vi "LM_I_27_07_16.vi"   [LabVIEW 2015]
uses:
  <vilib>/NXT/Block Support/NXT_MessageMailbox.ctl
  <vilib>/NXT/Block Support/NXT_OutputPort.ctl
  <vilib>/NXT/Subs/MotorOutput.ctl
  <vilib>/NXT/Block Support/NXT_InputPort.ctl
  <vilib>/NXT/Block Support/NXT_TimerIndex.ctl
  <vilib>/NXT/Dual Mode Library/Advanced/NXTFlag_Assign.vi
  <vilib>/NXT/NXTIO Xnodes/NXTIONodeSubVIs/NXTMoveMotors.vi
  <vilib>/NXT/NXTIO Xnodes/NXTIONodeSubVIs/NXTStopMotors.vi
  <vilib>/NXT/Dual Mode Library/BT/BlueTooth_Write_String.vi
  <vilib>/NXT/Subs/LVHSConnector.ctl
  <vilib>/NXT/NXTIO Xnodes/AddressXNode/NXTIOAddress.xnode
  <vilib>/NXT/NXTIO Xnodes/NXTIOXNode/NXTIO.xnode
  <vilib>/NXT/LegoClasses/BrickReference/BrickReference.lvclass
types:
  T1 = typedef "NXT_MessageMailbox.ctl" = u8
  T2 = typedef "LVHSConnector.ctl" = refnum<class "BrickReference.lvclass">
  T3 = typedef "NXT_InputPort.ctl" = u32
  T4 = typedef "NXT_OutputPort.ctl" = u8
  T5 = typedef "NXT_TimerIndex.ctl" = u8
  T6 = typedef "MotorOutput.ctl" = u8
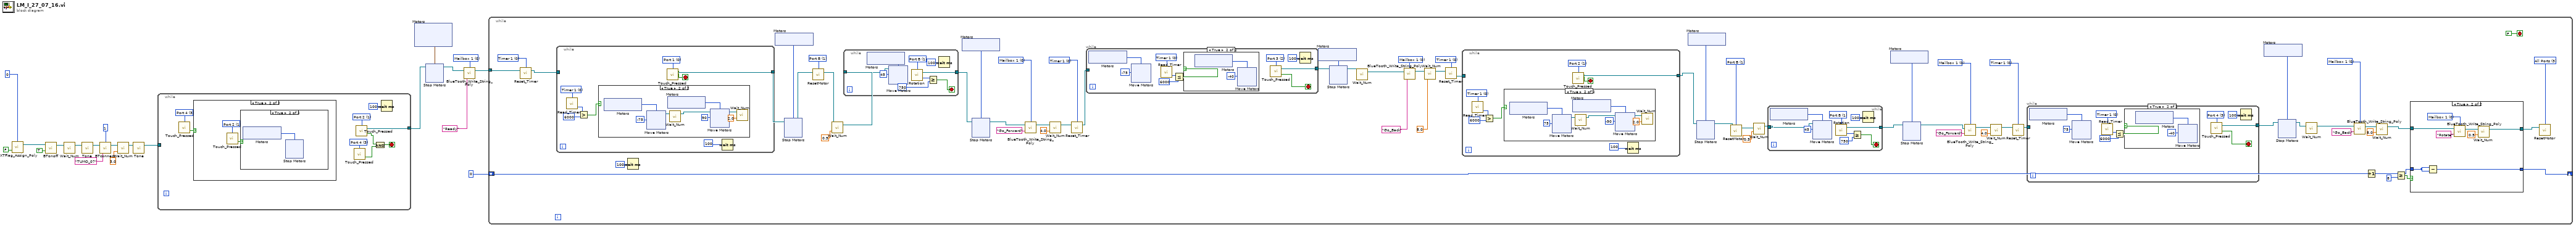
[diagram p0: block diagram]
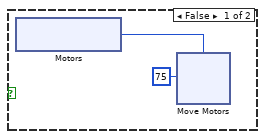
[diagram p2: hidden frame]
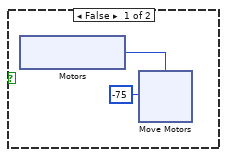
[diagram p3: hidden frame]
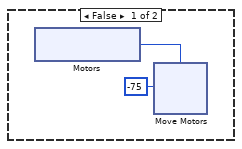
[diagram p4: hidden frame]
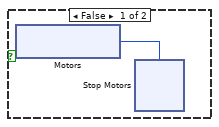
[diagram p5: hidden frame]
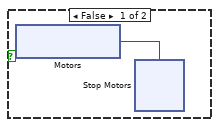
[diagram p7: hidden frame]
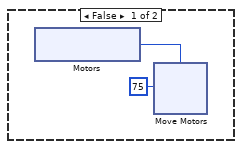
[diagram p8: hidden frame]
diagram:
  w8 = T1 0 items=["Mailbox 1", "Mailbox 2", "Mailbox 3", "Mailbox 4", "Mailbox 5", "Mailbox 6", "Mailbox 7", "Mailbox 8", "Mailbox 9", "Mailbox 10"] ("Mailbox")
  n1 = call-poly <vilib>:"NXTFlag_Assign_Poly.vi"("Flag State"=FALSE, "NXT/EV3 Flag Number"=i8 0) -> ("NXT/EV3"=w4:T2)  [unwired: 2 in]
  n2 = call <vilib>:"BTonoff.vi"("On/Off"=TRUE, "NXT/EV3"=w4) -> ("NXT/EV3"=w13:T2)  [unwired: 1 in, 1 out]
  n3 = call <vilib>:"Wait_Num.vi"("NXT/EV3"=w13) -> ("NXT/EV3"=w12:T2)  [unwired: 3 in]
  n4 = call <vilib>:"Tone.vi"("NXT/EV3"=w12) -> ("NXT/EV3"=w11:T2)  [unwired: 3 in]
  n5 = call <vilib>:"BTconnect.vi"("Partner Name"="TUMO_07", "NXT/EV3"=w11, "Connection"=u8 1) -> ("NXT/EV3"=w19:T2)  [unwired: 1 out]
  n6 = call <vilib>:"Wait_Num.vi"("Time (1 sec)"=sgl 3.0, "NXT/EV3"=w19) -> ("NXT/EV3"=w14:T2)  [unwired: 2 in]
  n7 = call <vilib>:"Tone.vi"("NXT/EV3"=w14) -> ("NXT/EV3"=w10:T2)  [unwired: 3 in]
  n8 = while {
    tunnel: w10 -> [_]
    tunnel: [w23] -> w6
    stop <- w27 stop-if-true
    w24 = T3 3 items=["Port 1", "Port 2", "Port 3", "Port 4"] ("Port (Port 1)")
    w28 = T3 3 items=["Port 1", "Port 2", "Port 3", "Port 4"] ("Port (Port 1)")
    w29 = T3 1 items=["Port 1", "Port 2", "Port 3", "Port 4"] ("Port (Port 1)")
    n9 = call <vilib>:"Touch_Pressed.vi"("Port (Port 1)"=w24) -> ("Yes / No"=w25:bool)  [unwired: 2 in, 1 out]
    n10 = case shown="True" w25 {
      frame False {
        n11 = xnode "Motors"() -> ("Motor"=w31:T4)
        n12 = xnode "Move Motors"("Power/Speed 1"=i8 75, "Motors"=w31) -> ()  [unwired: 1 in, 1 out]
      }
      frame True {
        w41 = T3 1 items=["Port 1", "Port 2", "Port 3", "Port 4"] ("Port (Port 1)")
        n13 = call <vilib>:"Touch_Pressed.vi"("Port (Port 1)"=w41) -> ("Yes / No"=w40:bool)  [unwired: 2 in, 1 out]
        n14 = case shown="True" w40 {
          frame False {
            n15 = xnode "Motors"() -> ("Motor"=w43:T4)
            n16 = xnode "Move Motors"("Power/Speed 1"=i8 -75, "Motors"=w43) -> ()  [unwired: 1 in, 1 out]
          }
          frame True {
            n17 = xnode "Motors"() -> ("Motor"=w52:T4)
            n18 = xnode "Stop Motors"("Motors"=w52) -> ()  [unwired: 1 in, 1 out]
          }
        }
      }
    }
    n19 = call <vilib>:"Touch_Pressed.vi"("Port (Port 1)"=w28) -> ("Yes / No"=w21:bool)  [unwired: 2 in, 1 out]
    n20 = call <vilib>:"Touch_Pressed.vi"("Port (Port 1)"=w29) -> ("Yes / No"=w22:bool, "NXT/EV3"=w23:T2)  [unwired: 2 in]
    n21 = And(x=w22, y=w21) -> (x .and. y?=w27:bool)
    n22 = Wait (ms)(milliseconds to wait=u32 100) -> ()  [unwired: 1 out]
  }
  n23 = xnode "Motors"() -> ("Motor"=w1:cluster{"Port":T4, "Port":T4, "Port":T4})
  n24 = xnode "Stop Motors"("Motors"=w1, "NXT/EV3"=w6) -> ("NXT/EV3"=w7:T2)
  n25 = call-poly <vilib>:"BlueTooth_Write_String_Poly.vi"("Message"="Ready", "NXT/EV3"=w7, "Mailbox"=w8) -> ("NXT/EV3"=w5:T2)  [unwired: 1 in]
  n26 = while {
    shift-right: [w87] -> _
    shift-left: u32 0 ("milliseconds to wait") -> [w66]
    tunnel: w5 -> [w65]
    stop <- FALSE stop-if-true
    w62 = T5 0 items=["Timer 1", "Timer 2", "Timer 3"] ("Timer (Timer 1)")
    w63 = T5 0 items=["Timer 1", "Timer 2", "Timer 3"] ("Timer (Timer 1)")
    w73 = T6 3 items=["Port A"=0, "Port B"=1, "Port C"=2, "Ports A & B"=4, "Ports A & C"=5, "Ports B & C"=6, "All Ports"=3] ("Port (All Ports)")
    w79 = T5 0 items=["Timer 1", "Timer 2", "Timer 3"] ("Timer (Timer 1)")
    w83 = T5 0 items=["Timer 1", "Timer 2", "Timer 3"] ("Timer (Timer 1)")
    w117 = T6 1 items=["Port A"=0, "Port B"=1, "Port C"=2, "Ports A & B"=4, "Ports A & C"=5, "Ports B & C"=6, "All Ports"=3] ("Port (All Ports)")
    w103 = T1 0 items=["Mailbox 1", "Mailbox 2", "Mailbox 3", "Mailbox 4", "Mailbox 5", "Mailbox 6", "Mailbox 7", "Mailbox 8", "Mailbox 9", "Mailbox 10"] ("Mailbox")
    w101 = T1 0 items=["Mailbox 1", "Mailbox 2", "Mailbox 3", "Mailbox 4", "Mailbox 5", "Mailbox 6", "Mailbox 7", "Mailbox 8", "Mailbox 9", "Mailbox 10"] ("Mailbox")
    w97 = T1 0 items=["Mailbox 1", "Mailbox 2", "Mailbox 3", "Mailbox 4", "Mailbox 5", "Mailbox 6", "Mailbox 7", "Mailbox 8", "Mailbox 9", "Mailbox 10"] ("Mailbox")
    w91 = T1 0 items=["Mailbox 1", "Mailbox 2", "Mailbox 3", "Mailbox 4", "Mailbox 5", "Mailbox 6", "Mailbox 7", "Mailbox 8", "Mailbox 9", "Mailbox 10"] ("Mailbox")
    w89 = T6 1 items=["Port A"=0, "Port B"=1, "Port C"=2, "Ports A & B"=4, "Ports A & C"=5, "Ports B & C"=6, "All Ports"=3] ("Port (All Ports)")
    n27 = call <vilib>:"Reset_Timer.vi"("NXT/EV3"=w65, "Timer (Timer 1)"=w63) -> ("NXT/EV3"=w64:T2)  [unwired: 2 in]
    n28 = while {
      tunnel: [w322] -> w93
      tunnel: w64 -> [_]
      stop <- w321 stop-if-true
      w320 = T5 0 items=["Timer 1", "Timer 2", "Timer 3"] ("Timer (Timer 1)")
      w323 = T3 0 items=["Port 1", "Port 2", "Port 3", "Port 4"] ("Port (Port 1)")
      n29 = call <vilib>:"Read_Timer.vi"("Timer (Timer 1)"=w320) -> ("Value (msec)"=w317:u32)  [unwired: 2 in, 1 out]
      n30 = Greater?(x=w317, y=u32 6000) -> (0:w319:bool)
      n31 = case shown="True" w319 {
        frame False {
          n32 = xnode "Motors"() -> ("Motor"=w325:T4)
          n33 = xnode "Move Motors"("Power/Speed 1"=i8 75, "Motors"=w325) -> ()  [unwired: 1 in, 1 out]
        }
        frame True {
          n34 = xnode "Motors"() -> ("Motor"=w341:T4)
          n35 = xnode "Move Motors"("Power/Speed 1"=i8 -75, "Motors"=w341) -> ("NXT/EV3"=w340:T2)  [unwired: 1 in]
          n36 = xnode "Motors"() -> ("Motor"=w338:T4)
          n37 = call <vilib>:"Wait_Num.vi"("NXT/EV3"=w340) -> ("NXT/EV3"=w337:T2)  [unwired: 3 in]
          n38 = xnode "Move Motors"("Power/Speed 1"=i8 90, "Motors"=w338, "NXT/EV3"=w337) -> ("NXT/EV3"=w336:T2)
          n39 = call <vilib>:"Wait_Num.vi"("Time (1 sec)"=sgl 2.0, "NXT/EV3"=w336) -> ()  [unwired: 2 in, 1 out]
        }
      }
      n40 = call <vilib>:"Touch_Pressed.vi"("Port (Port 1)"=w323) -> ("Yes / No"=w321:bool, "NXT/EV3"=w322:T2)  [unwired: 2 in]
      n41 = Wait (ms)(milliseconds to wait=u32 100) -> ()  [unwired: 1 out]
    }
    n42 = Wait (ms)(milliseconds to wait=u32 100) -> ()  [unwired: 1 out]
    n43 = xnode "Motors"() -> ("Motor"=w72:T4)
    n44 = xnode "Stop Motors"("Motors"=w72, "NXT/EV3"=w93) -> ("NXT/EV3"=w92:T2)
    n45 = call <vilib>:"ResetMotor.vi"("NXT/EV3"=w92, "Port (All Ports)"=w89) -> ("NXT/EV3"=w114:T2)  [unwired: 2 in]
    n46 = call <vilib>:"Wait_Num.vi"("Time (1 sec)"=sgl 0.5, "NXT/EV3"=w114) -> ("NXT/EV3"=w115:T2)  [unwired: 2 in]
    n47 = while {
      tunnel: w115 -> [w308]
      tunnel: [w305] -> w94
      stop <- w301 stop-if-true
      w307 = T6 1 items=["Port A"=0, "Port B"=1, "Port C"=2, "Ports A & B"=4, "Ports A & C"=5, "Ports B & C"=6, "All Ports"=3] ("Output Port (All Ports)")
      n48 = xnode "Motors"() -> ("Motor"=w303:T4)
      n49 = xnode "Move Motors"("Power/Speed 1"=i8 45, "Motors"=w303, "NXT/EV3"=w308) -> ()  [unwired: 1 out]
      n50 = call <vilib>:"Rotation.vi"("Port (Port A)"=w307) -> ("Angle of Rotation"=w300:i32, "NXT/EV3"=w305:T2)  [unwired: 2 in]
      n51 = Greater Or Equal?(x=w300, y=750) -> (x >= y?=w301:bool)
      n52 = Wait (ms)(milliseconds to wait=u32 100) -> ()  [unwired: 1 out]
    }
    n53 = xnode "Motors"() -> ("Motor"=w71:T4)
    n54 = xnode "Stop Motors"("Motors"=w71, "NXT/EV3"=w94) -> ("NXT/EV3"=w95:T2)
    n55 = call-poly <vilib>:"BlueTooth_Write_String_Poly.vi"("Message"="Go_Forward", "NXT/EV3"=w95, "Mailbox"=w91) -> ("NXT/EV3"=w86:T2)  [unwired: 1 in]
    n56 = call <vilib>:"Wait_Num.vi"("Time (1 sec)"=sgl 4.0, "NXT/EV3"=w86) -> ("NXT/EV3"=w84:T2)  [unwired: 2 in]
    n57 = call <vilib>:"Reset_Timer.vi"("NXT/EV3"=w84, "Timer (Timer 1)"=w83) -> ("NXT/EV3"=w82:T2)  [unwired: 2 in]
    n58 = while {
      tunnel: w82 -> [_]
      tunnel: [w268] -> w81
      stop <- w265 stop-if-true
      w269 = T5 0 items=["Timer 1", "Timer 2", "Timer 3"] ("Timer (Timer 1)")
      w274 = T3 2 items=["Port 1", "Port 2", "Port 3", "Port 4"] ("Port (Port 1)")
      n59 = xnode "Motors"() -> ("Motor"=w267:T4)
      n60 = xnode "Move Motors"("Power/Speed 1"=i8 -75, "Motors"=w267) -> ()  [unwired: 1 in, 1 out]
      n61 = call <vilib>:"Read_Timer.vi"("Timer (Timer 1)"=w269) -> ("Value (msec)"=w272:u32)  [unwired: 2 in, 1 out]
      n62 = Less Or Equal?(x=w272, y=u32 6000) -> (x <= y?=w270:bool)
      n63 = case shown="True" w270 {
        frame False {
          n64 = xnode "Motors"() -> ("Motor"=w283:T4)
          n65 = xnode "Stop Motors"("Motors"=w283) -> ()  [unwired: 1 in, 1 out]
        }
        frame True {
          n66 = xnode "Motors"() -> ("Motor"=w291:T4)
          n67 = xnode "Move Motors"("Power/Speed 1"=i8 -40, "Motors"=w291) -> ()  [unwired: 1 in, 1 out]
        }
      }
      n68 = call <vilib>:"Touch_Pressed.vi"("Port (Port 1)"=w274) -> ("Yes / No"=w265:bool, "NXT/EV3"=w268:T2)  [unwired: 2 in]
      n69 = Wait (ms)(milliseconds to wait=u32 100) -> ()  [unwired: 1 out]
    }
    n70 = xnode "Motors"() -> ("Motor"=w70:T4)
    n71 = xnode "Stop Motors"("Motors"=w70, "NXT/EV3"=w81) -> ("NXT/EV3"=w110:T2)
    n72 = call <vilib>:"Wait_Num.vi"("NXT/EV3"=w110) -> ("NXT/EV3"=w111:T2)  [unwired: 3 in]
    n73 = call-poly <vilib>:"BlueTooth_Write_String_Poly.vi"("Message"="Go_Back", "NXT/EV3"=w111, "Mailbox"=w97) -> ("NXT/EV3"=w98:T2)  [unwired: 1 in]
    n74 = call <vilib>:"Wait_Num.vi"("Time (1 sec)"=sgl 8.0, "NXT/EV3"=w98) -> ("NXT/EV3"=w60:T2)  [unwired: 2 in]
    n75 = call <vilib>:"Reset_Timer.vi"("NXT/EV3"=w60, "Timer (Timer 1)"=w62) -> ("NXT/EV3"=w61:T2)  [unwired: 2 in]
    n76 = while {
      tunnel: [w130] -> w59
      tunnel: w61 -> [_]
      stop <- w129 stop-if-true
      w128 = T5 0 items=["Timer 1", "Timer 2", "Timer 3"] ("Timer (Timer 1)")
      w131 = T3 1 items=["Port 1", "Port 2", "Port 3", "Port 4"] ("Port (Port 1)")
      n77 = call <vilib>:"Read_Timer.vi"("Timer (Timer 1)"=w128) -> ("Value (msec)"=w125:u32)  [unwired: 2 in, 1 out]
      n78 = Greater?(x=w125, y=u32 6000) -> (0:w127:bool)
      n79 = case shown="True" w127 {
        frame False {
          n80 = xnode "Motors"() -> ("Motor"=w133:T4)
          n81 = xnode "Move Motors"("Power/Speed 1"=i8 -75, "Motors"=w133) -> ()  [unwired: 1 in, 1 out]
        }
        frame True {
          n82 = xnode "Motors"() -> ("Motor"=w149:T4)
          n83 = xnode "Move Motors"("Power/Speed 1"=i8 75, "Motors"=w149) -> ("NXT/EV3"=w148:T2)  [unwired: 1 in]
          n84 = xnode "Motors"() -> ("Motor"=w146:T4)
          n85 = call <vilib>:"Wait_Num.vi"("NXT/EV3"=w148) -> ("NXT/EV3"=w145:T2)  [unwired: 3 in]
          n86 = xnode "Move Motors"("Power/Speed 1"=i8 -90, "Motors"=w146, "NXT/EV3"=w145) -> ("NXT/EV3"=w144:T2)
          n87 = call <vilib>:"Wait_Num.vi"("Time (1 sec)"=sgl 2.0, "NXT/EV3"=w144) -> ()  [unwired: 2 in, 1 out]
        }
      }
      n88 = call <vilib>:"Touch_Pressed.vi"("Port (Port 1)"=w131) -> ("Yes / No"=w129:bool, "NXT/EV3"=w130:T2)  [unwired: 2 in]
      n89 = Wait (ms)(milliseconds to wait=u32 100) -> ()  [unwired: 1 out]
    }
    n90 = xnode "Motors"() -> ("Motor"=w69:T4)
    n91 = xnode "Stop Motors"("Motors"=w69, "NXT/EV3"=w59) -> ("NXT/EV3"=w121:T2)
    n92 = call <vilib>:"ResetMotor.vi"("NXT/EV3"=w121, "Port (All Ports)"=w117) -> ("NXT/EV3"=w122:T2)  [unwired: 2 in]
    n93 = call <vilib>:"Wait_Num.vi"("Time (1 sec)"=sgl 0.5, "NXT/EV3"=w122) -> ("NXT/EV3"=w123:T2)  [unwired: 2 in]
    n94 = while {
      tunnel: [w244] -> w118
      tunnel: w123 -> [w242]
      stop <- w246 stop-if-true
      w243 = T4 1 items=["Port A", "Port B", "Port C", "Port D"] ("Port (Port A)")
      n95 = xnode "Motors"() -> ("Motor"=w240:T4)
      n96 = xnode "Move Motors"("Power/Speed 1"=i8 45, "Motors"=w240, "NXT/EV3"=w242) -> ()  [unwired: 1 out]
      n97 = call <vilib>:"Rotation.vi"("Port (Port A)"=w243) -> ("Angle of Rotation"=w238:i32, "NXT/EV3"=w244:T2)  [unwired: 2 in]
      n98 = Greater Or Equal?(x=w238, y=750) -> (x >= y?=w246:bool)
      n99 = Wait (ms)(milliseconds to wait=u32 100) -> ()  [unwired: 1 out]
    }
    n100 = xnode "Motors"() -> ("Motor"=w68:T4)
    n101 = xnode "Stop Motors"("Motors"=w68, "NXT/EV3"=w118) -> ("NXT/EV3"=w120:T2)
    n102 = call-poly <vilib>:"BlueTooth_Write_String_Poly.vi"("Message"="Go_Forward", "NXT/EV3"=w120, "Mailbox"=w101) -> ("NXT/EV3"=w76:T2)  [unwired: 1 in]
    n103 = call <vilib>:"Wait_Num.vi"("Time (1 sec)"=sgl 4.0, "NXT/EV3"=w76) -> ("NXT/EV3"=w78:T2)  [unwired: 2 in]
    n104 = call <vilib>:"Reset_Timer.vi"("NXT/EV3"=w78, "Timer (Timer 1)"=w79) -> ("NXT/EV3"=w80:T2)  [unwired: 2 in]
    n105 = while {
      tunnel: w80 -> [_]
      tunnel: [w206] -> w75
      stop <- w203 stop-if-true
      w207 = T5 0 items=["Timer 1", "Timer 2", "Timer 3"] ("Timer (Timer 1)")
      w212 = T3 3 items=["Port 1", "Port 2", "Port 3", "Port 4"] ("Port (Port 1)")
      n106 = xnode "Motors"() -> ("Motor"=w205:T4)
      n107 = xnode "Move Motors"("Power/Speed 1"=i8 75, "Motors"=w205) -> ()  [unwired: 1 in, 1 out]
      n108 = call <vilib>:"Read_Timer.vi"("Timer (Timer 1)"=w207) -> ("Value (msec)"=w210:u32)  [unwired: 2 in, 1 out]
      n109 = Less Or Equal?(x=w210, y=u32 6000) -> (x <= y?=w208:bool)
      n110 = case shown="True" w208 {
        frame False {
          n111 = xnode "Motors"() -> ("Motor"=w221:T4)
          n112 = xnode "Stop Motors"("Motors"=w221) -> ()  [unwired: 1 in, 1 out]
        }
        frame True {
          n113 = xnode "Motors"() -> ("Motor"=w229:T4)
          n114 = xnode "Move Motors"("Power/Speed 1"=i8 -40, "Motors"=w229) -> ()  [unwired: 1 in, 1 out]
        }
      }
      n115 = call <vilib>:"Touch_Pressed.vi"("Port (Port 1)"=w212) -> ("Yes / No"=w203:bool, "NXT/EV3"=w206:T2)  [unwired: 2 in]
      n116 = Wait (ms)(milliseconds to wait=u32 100) -> ()  [unwired: 1 out]
    }
    n117 = xnode "Motors"() -> ("Motor"=w67:T4)
    n118 = xnode "Stop Motors"("Motors"=w67, "NXT/EV3"=w75) -> ("NXT/EV3"=w112:T2)
    n119 = call <vilib>:"Wait_Num.vi"("NXT/EV3"=w112) -> ("NXT/EV3"=w113:T2)  [unwired: 3 in]
    n120 = call-poly <vilib>:"BlueTooth_Write_String_Poly.vi"("Message"="Go_Back", "NXT/EV3"=w113, "Mailbox"=w103) -> ("NXT/EV3"=w104:T2)  [unwired: 1 in]
    n121 = Increment(x=w66) -> (x+1=w108:u32)
    n122 = call <vilib>:"Wait_Num.vi"("Time (1 sec)"=sgl 8.0, "NXT/EV3"=w104) -> ("NXT/EV3"=w109:T2)  [unwired: 2 in]
    n123 = Greater Or Equal?(x=w108, y=u32 8) -> (x >= y?=w107:bool)
    n124 = case shown="True" w107 {
      tunnel: w108 -> [w256 w264]
      tunnel: [w256 w258] -> w87
      tunnel: w109 -> [w255 w259]
      tunnel: [w255 w257] -> w74
      frame False {
      }
      frame True {
        w262 = T1 0 items=["Mailbox 1", "Mailbox 2", "Mailbox 3", "Mailbox 4", "Mailbox 5", "Mailbox 6", "Mailbox 7", "Mailbox 8", "Mailbox 9", "Mailbox 10"] ("Mailbox")
        n125 = Subtract(x=w264, y=w264) -> (x-y=w258:u32)
        n126 = call-poly <vilib>:"BlueTooth_Write_String_Poly.vi"("Message"="Rotate", "NXT/EV3"=w259, "Mailbox"=w262) -> ("NXT/EV3"=w261:T2)  [unwired: 1 in]
        n127 = call <vilib>:"Wait_Num.vi"("Time (1 sec)"=sgl 0.5, "NXT/EV3"=w261) -> ("NXT/EV3"=w257:T2)  [unwired: 2 in]
      }
    }
    n128 = call <vilib>:"ResetMotor.vi"("NXT/EV3"=w74, "Port (All Ports)"=w73) -> ()  [unwired: 2 in, 1 out]
  }
